vi "Hash-string.vi"(7 "HASH-method":T1=enum."SHA-256" caption="HASH-method (SHA-256)", 8 "error in (no error)":errorcluster, 11 "Message":u8[](array[numeric])) -> (0 "error out":errorcluster, 1 "ASCII formatted hash":string, 3 "Hash":u8[](array[numeric]))   [LabVIEW 2011, in "i3-external-encryption.lvlib"]
doc: "Calculates a hash for the given <b>Message</b>.\n\n(c) Ton Plomp, 2011\nTHIS SOFTWARE IS PROVIDED AS IS, AND ANY WARRANTY IS REJECTED"
uses:
  i3-external-encryption.lvlib
  hash-types.ctl
  SHA/SHA-2_U32_types.ctl
  SHA/SHA-2_U64_types.ctl
  <userlib>/_OpenG.lib/md5/md5.llb/MD5 Message Digest (Binary String)__ogtk.vi
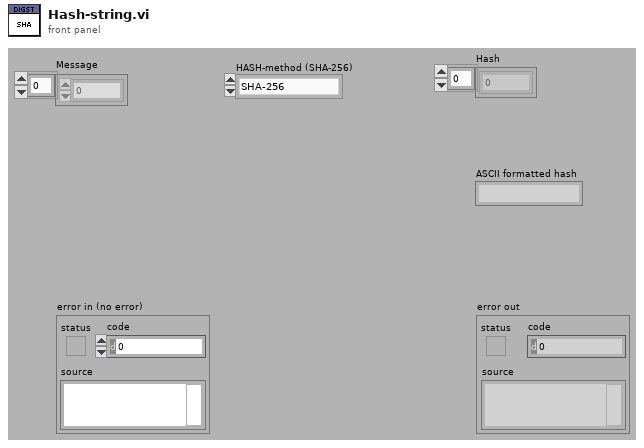
[diagram p1: front panel]
types:
  T1 = typedef "i3-external-encryption.lvlib/hash-types.ctl" = enum16{"MD5", "SHA-1", "SHA-224", "SHA-256", "SHA-384", "SHA-512"}
  T2 = typedef "i3-external-encryption.lvlib/SHA-2_U32_types.ctl" = enum16{"256", "224"}
  T3 = typedef "i3-external-encryption.lvlib/SHA-2_U64_types.ctl" = enum16{"512", "384"}
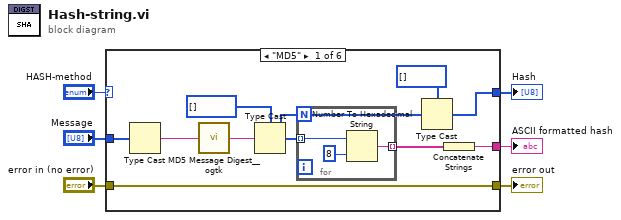
[diagram p0: block diagram]
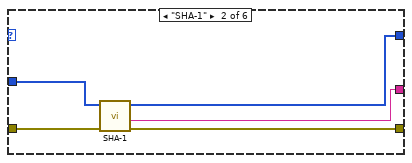
[diagram p2: hidden frame]
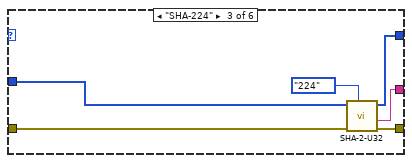
[diagram p3: hidden frame]
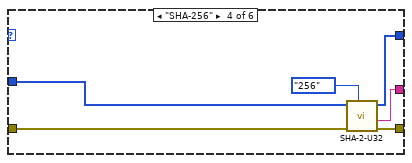
[diagram p4: hidden frame]
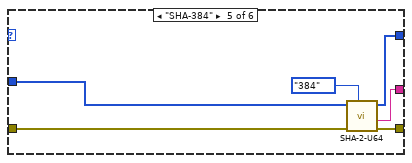
[diagram p5: hidden frame]
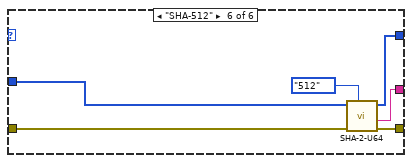
[diagram p6: hidden frame]
diagram:
  n1 = case shown="\"MD5\"" "HASH-method" {
    tunnel: "Message" -> [w10 w24 w30 w36 w42 w48]
    tunnel: [w13 w23 w29 w35 w41 w47] -> w4
    tunnel: "error in (no error)" -> [w13 w22 w28 w34 w40 w46]
    tunnel: [w7 w21 w27 w33 w39 w45] -> w2
    tunnel: [w14 w20 w26 w32 w38 w44] -> w1
    frame "MD5" {
      n2 = Type Cast(x=w10) -> (*(type *) &x=w11:string)  [unwired: 1 in]
      n3 = call-poly <userlib>:"MD5 Message Digest__ogtk.vi"("Message"=w11) -> ("MD5 Message Digest"=w15:string)
      n4 = Type Cast(type=u32[] [], x=w15) -> (*(type *) &x=w8:u32[])
      n5 = for {
        tunnel: w8 -> [w19] mode=indexing
        tunnel: [w17] -> w16 mode=indexing
        n6 = Number To Hexadecimal String(1:i16 8 ("width (-)"), 2:w19) -> (0:w17:string)
      }
      n7 = Type Cast(type=u8[] [] ("binary string hash"), x=w8) -> (*(type *) &x=w7:u8[])
      n8 = Concatenate Strings(w16) -> (w14:string)
    }
    frame "SHA-1" {
      n9 = call "SHA-1.vi"("error in (no error)"=w22, "Message"=w24) -> ("error out"=w23:errorcluster, "ASCII Formatted hash"=w20:string, "Hash"=w21:u8[])  [unwired: 7 in]
    }
    frame "SHA-224" {
      n10 = call "SHA-2-U32.vi"("Type"=SHA-2_U32_types."224", "error in (no error)"=w28, "Message"=w30) -> ("error out"=w29:errorcluster, "ASCII formatted hash"=w26:string, "Hash"=w27:u8[])  [unwired: 6 in]
    }
    frame "SHA-256" {
      n11 = call "SHA-2-U32.vi"("Type"=SHA-2_U32_types."256", "error in (no error)"=w34, "Message"=w36) -> ("error out"=w35:errorcluster, "ASCII formatted hash"=w32:string, "Hash"=w33:u8[])  [unwired: 6 in]
    }
    frame "SHA-384" {
      n12 = call "SHA-2-U64.vi"("Type"=SHA-2_U64_types."384", "error in (no error)"=w40, "Message"=w42) -> ("error out"=w41:errorcluster, "ASCII Formatted hash"=w38:string, "binary string hash"=w39:u8[])  [unwired: 6 in]
    }
    frame "SHA-512" {
      n13 = call "SHA-2-U64.vi"("Type"=SHA-2_U64_types."512", "error in (no error)"=w46, "Message"=w48) -> ("error out"=w47:errorcluster, "ASCII Formatted hash"=w44:string, "binary string hash"=w45:u8[])  [unwired: 6 in]
    }
  }
  "error out" <- w4
  "Hash" <- w2
  "ASCII formatted hash" <- w1
